vi "Read ID.vi"(8 "error in (no error)":errorcluster, 11 "Simulated in":refnum<class "Simulated.lvclass">) -> (0 "error out":errorcluster, 2 "ID":string, 3 "Simulated out":refnum<class "Simulated.lvclass">)   [LabVIEW 2016, in "Simulated.lvclass"]
uses:
  Simulated.lvclass
  Parent/Hardware.lvclass
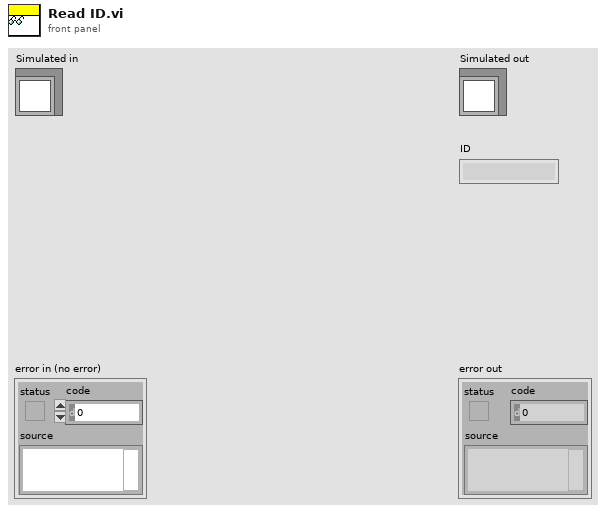
[diagram p1: front panel]
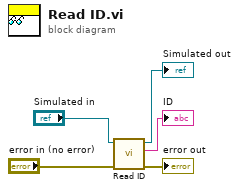
[diagram p0: block diagram]
diagram:
  n1 = call-parent "Read ID.vi"("error in (no error)"="error in (no error)", "Hardware in"="Simulated in") -> ("error out"=→"error out":errorcluster, "ID"=→"ID":string, "Hardware out"=→"Simulated out":refnum<class "Simulated.lvclass">)  [unwired: 7 in]
